vi "get Spectra.vi"() -> ()   [LabVIEW 2020, in "FT-IR.lvlib" / "Get Spectra.lvlib"]
uses:
  Get Spectra.lvlib
  FTIR Diag.ctl
  Aktion FGV Background-Daten.ctl
  FGV FT-IR Diagnose Aktionen.ctl
  Allgemein/allgemeine Sub-VIs.lvlib
  FT-IR.lvlib
panel:
  out "Zeitstempel GB":timestamp caption="Timestamp GoldenBackground" format="%<%x>T"
  in  "GoldenBackground erzeugen":bool caption="Stopp"
  out "DiagLabels":string[](array[string])=["igramdc", "igrampp", "phaseAngle", "laserpp", "laserdc", "badscan", "centerburst", "linCheck", "sBeamIntensity"]
  out "Diagnosewerte für Backup":sgl[](array[numeric])
  out "Zeitstempel":timestamp caption="Timestamp Reference"
  in  "Referenz":bool
  in  "@2500":bool
  in  "FTIR Diag":T1 items=["Background Igram", "Background sBeam", "sample Igram", "sample Background", "sample Absorbance"]
  out "XY-Graph":cluster{"Ramp Pattern":dbl[], dbl[]}[](graph)
  in  "Stopp":bool
  # "FT-IR Diagnose"
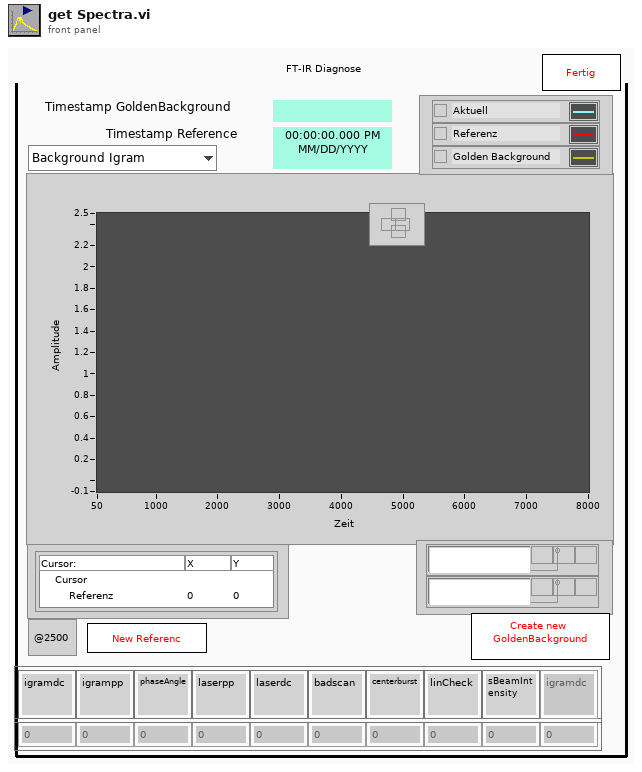
[diagram p1: front panel]
types:
  T1 = typedef "FT-IR.lvlib/Get Spectra.lvlib/FTIR Diag.ctl" = u16
  T2 = typedef "FT-IR.lvlib/Get Spectra.lvlib/Aktion FGV Background-Daten.ctl" = enum16{"lesen", "schreiben", "Background aktiv", "Referenz", "laden", "speichern", "Plot sichtbar"}
  T3 = typedef "FT-IR.lvlib/FGV FT-IR Diagnose Aktionen.ctl" = enum16{"Lesen", "Diagnose Schreiben", "Min Schreiben", "Max Schreiben"}
  T4 = typedef "FT-IR.lvlib/TOOLweb Interface.lvlib/Typdefinitionen.lvlib/TOOLweb Diagnose.ctl" = cluster{"(14) temperature":sgl, "(15) pressure":sgl, "(16) oxygen":sgl, "(50) diag-igramdc":sgl, "(51) diag-igrampp":sgl, "(52) diag-phaseAngle":sgl, "(53) diag-laserpp":sgl, "(54) diag-laserdc":sgl, "(55) diag-badscan":sgl, "(56) diag-centerburst":sgl, "(57) diag-linearizerCheck":sgl, "(58) diag-SNR":sgl, "(59) diag-sBeamIntensity":sgl}
  T5 = typedef "LVPositionTypeDef.ctl" = cluster{"Left":i32, "Top":i32}
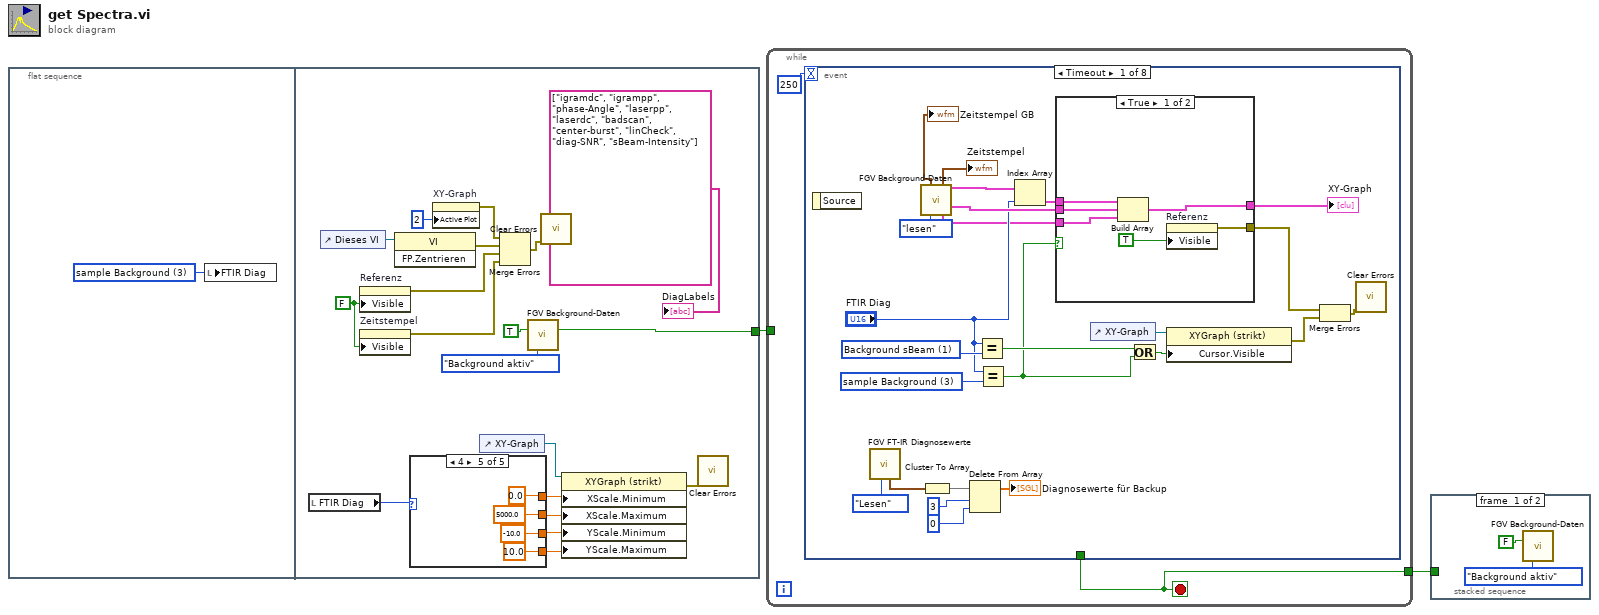
[diagram p0: block diagram]
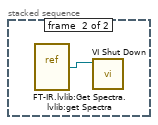
[diagram p2: hidden frame]
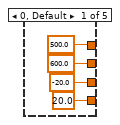
[diagram p3: hidden frame]
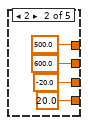
[diagram p4: hidden frame]
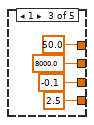
[diagram p5: hidden frame]
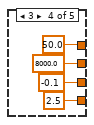
[diagram p6: hidden frame]
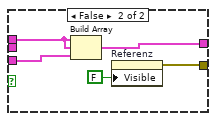
[diagram p7: hidden frame]
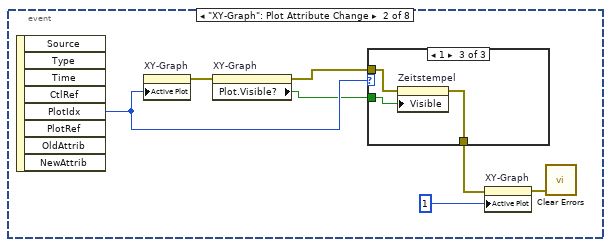
[diagram p8: hidden frame]
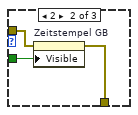
[diagram p10: hidden frame]
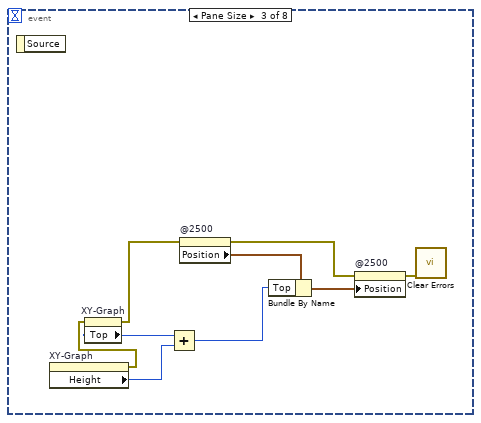
[diagram p11: hidden frame]
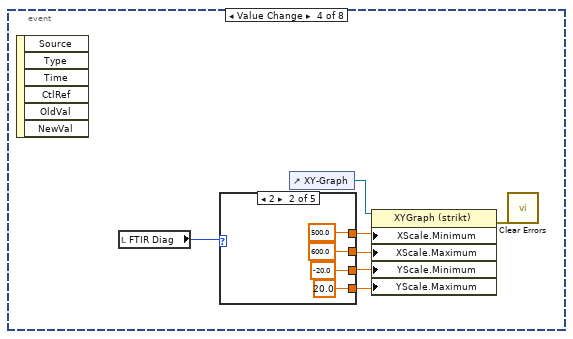
[diagram p12: hidden frame]
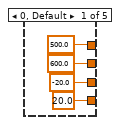
[diagram p13: hidden frame]
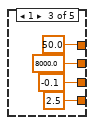
[diagram p14: hidden frame]
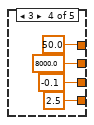
[diagram p15: hidden frame]
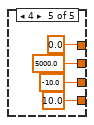
[diagram p16: hidden frame]
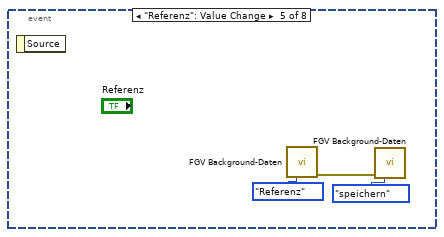
[diagram p17: hidden frame]
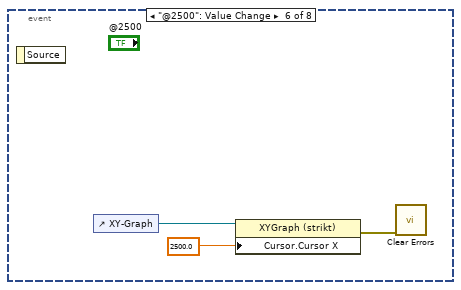
[diagram p18: hidden frame]
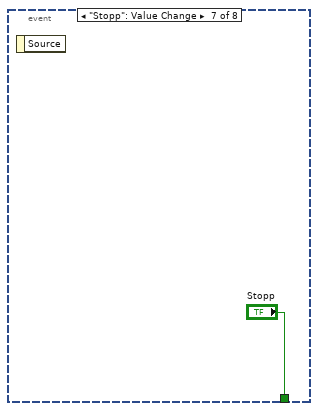
[diagram p19: hidden frame]
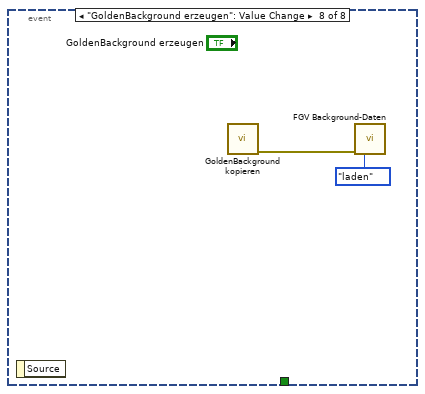
[diagram p20: hidden frame]
diagram:
  n1 = flat-sequence {
    tunnel: [w20] -> w1
    frame #0 {
      w3 = T1 3 items=["Background Igram", "Background sBeam", "sample Igram", "sample Background", "sample Absorbance"] ("FTIR Diag")
      n2 = local write "FTIR Diag"(w3) -> ()
    }
    frame #1 {
      w13 = FALSE ("Sichtbar")
      n3 = local read "FTIR Diag"() -> (w5:T1)
      n4 = control-ref of="Dieses VI"() -> (w19:refnum<vi>)
      n5 = property on="Referenz" class="Bool."("Visible"=w13) -> (error out=w14:errorcluster)  [unwired: 2 in, 1 out]
      n6 = property on="Zeitstempel" class="AbsZeit (strikt)"("Visible"=w13) -> (error out=w12:errorcluster)  [unwired: 2 in, 1 out]
      n7 = invoke class="VI" method="FP.Zentrieren"(reference=w19) -> (error out=w17:errorcluster)  [unwired: 2 in, 2 out]
      n8 = case shown="4" w5 {
        tunnel: [500.0 ("X-Achse.Bereich:Minimum") 500.0 ("X-Achse.Bereich:Minimum") 50.0 ("X-Achse.Bereich:Minimum") 50.0 ("X-Achse.Bereich:Minimum") 0.0 ("X-Achse.Bereich:Minimum")] -> w9
        tunnel: [600.0 ("X-Achse.Bereich:Minimum") 600.0 ("X-Achse.Bereich:Minimum") 8000.0 ("X-Achse.Bereich:Minimum") 8000.0 ("X-Achse.Bereich:Minimum") 5000.0 ("X-Achse.Bereich:Minimum")] -> w8
        tunnel: [-20.0 ("X-Achse.Bereich:Minimum") -20.0 ("X-Achse.Bereich:Minimum") -0.1 ("X-Achse.Bereich:Minimum") -0.1 ("X-Achse.Bereich:Minimum") -10.0 ("X-Achse.Bereich:Minimum")] -> w10
        tunnel: [20.0 ("X-Achse.Bereich:Minimum") 20.0 ("X-Achse.Bereich:Minimum") 2.5 ("X-Achse.Bereich:Minimum") 2.5 ("X-Achse.Bereich:Minimum") 10.0 ("X-Achse.Bereich:Minimum")] -> w11
        frame 0, Default {
        }
        frame 2 {
        }
        frame 1 {
        }
        frame 3 {
        }
        frame 4 {
        }
      }
      n9 = property on="XY-Graph" class="XYGraph (strikt)"("Active Plot"=u32 2 ("Aktiver Plot")) -> (error out=w16:errorcluster)  [unwired: 2 in, 1 out]
      n10 = control-ref of="XY-Graph"() -> (w7:refnum<vi>)
      n11 = Merge Errors(w16, w17, w14, w12) -> (w15:errorcluster)
      n12 = call "FGV Background-Daten.vi"("Background aktiv"=TRUE, "Aktion"=Aktion_FGV_Background-Daten."Background aktiv") -> ("Background aktiv"=w20:bool)  [unwired: 6 in, 7 out]
      n13 = call <vilib>:"Clear Errors.vi"("error in (no error)"=w15) -> ()  [unwired: 5 in, 2 out]
      n14 = property class="XYGraph (strikt)"(reference=w7, "XScale.Minimum"=w9, "XScale.Maximum"=w8, "YScale.Minimum"=w10, "YScale.Maximum"=w11) -> (error out=w6:errorcluster)  [unwired: 1 in, 1 out]
      n15 = call <vilib>:"Clear Errors.vi"("error in (no error)"=w6) -> ()  [unwired: 5 in, 2 out]
      "DiagLabels" <- string[] ["igramdc", "igrampp", "phase-Angle", "laserpp", "laserdc", "badscan", "center-burst", "linCheck", "diag-SNR", "sBeam-Intensity"]
    }
  }
  n16 = while {
    tunnel: [w43] -> w2
    tunnel: w1 -> [_]
    stop <- w43 stop-if-true
    n17 = event shown="[0] Timeout" {
      selector: _ -> [_ _ _ _ _ _ _ _]
      dyn-events: _ -> [_ _ _ _ _ _ _ _]
      timeout: 250 -> [_ _ _ _ _ _ _ _]
      tunnel: [_ _ _ _ _ _ "Stopp" _] -> w43
      event Timeout {
        w64 = T1 3 items=["Background Igram", "Background sBeam", "sample Igram", "sample Background", "sample Absorbance"] ("y")
        w65 = T1 1 items=["Background Igram", "Background sBeam", "sample Igram", "sample Background", "sample Absorbance"] ("y")
        n18 = event-data() -> ()  [unwired: 1 in, 1 out]
        n19 = call "FGV FT-IR Diagnosewerte.vi"("Aktionen"=FGV_FT-IR_Diagnose_Aktionen."Lesen") -> ("Diagnose mean"=w47:T4)  [unwired: 5 in, 5 out]
        n20 = call "FGV Background-Daten.vi"("Aktion"=Aktion_FGV_Background-Daten."lesen") -> ("Zeitstempel GB"=→"Zeitstempel GB":timestamp, "Zeitstempel"=→"Zeitstempel":timestamp, "Background Daten"=w67:cluster{"Ramp Pattern":dbl[], dbl[]}[], "Referenz"=w60:cluster{"Ramp Pattern":dbl[], dbl[]}, "Golden Background"=w46:cluster{dbl[], "[Y]":sgl[]})  [unwired: 7 in, 3 out]
        n21 = Cluster To Array(cluster=w47) -> (array=w51:sgl[])
        n22 = Delete From Array(array=w51, length=3 ("Länge"), index=0 ("Index")) -> (array with subset deleted=→"Diagnosewerte für Backup":sgl[])  [unwired: 1 out]
        n23 = Equal?(x="FTIR Diag", y=w65) -> (x = y?=w63:bool)
        n24 = Equal?(x="FTIR Diag", y=w64) -> (x = y?=w58:bool)
        n25 = Index Array(array=w67, index="FTIR Diag") -> (element=w61:cluster{"Ramp Pattern":dbl[], dbl[]})
        n26 = case shown="True" w58 {
          tunnel: w61 -> [w74 w78]
          tunnel: w60 -> [w73 _]
          tunnel: [w72 w79] -> w59
          tunnel: [w71 w77] -> w55
          tunnel: w46 -> [w69 w75]
          frame True {
            n27 = Build Array(w74, w73, w69) -> (w72:cluster{"Ramp Pattern":dbl[], "[Y]":dbl[]}[])
            n28 = property on="Referenz" class="Bool."("Visible"=TRUE ("Sichtbar")) -> (error out=w71:errorcluster)  [unwired: 2 in, 1 out]
          }
          frame False {
            n29 = Build Array(w78, w78, w75) -> (w79:cluster{"Ramp Pattern":dbl[], "[Y]":dbl[]}[])
            n30 = property on="Referenz" class="Bool."("Visible"=FALSE ("Sichtbar")) -> (error out=w77:errorcluster)  [unwired: 2 in, 1 out]
          }
        }
        "XY-Graph" <- w59
        n31 = control-ref of="XY-Graph"() -> (w66:refnum<vi>)
        n32 = Or(x=w63, y=w58) -> (x .or. y?=w62:bool)
        n33 = property class="XYGraph (strikt)"(reference=w66, "Cursor.Visible"=w62) -> (error out=w57:errorcluster)  [unwired: 1 in, 1 out]
        n34 = Merge Errors(w55, w57) -> (w56:errorcluster)
        n35 = call <vilib>:"Clear Errors.vi"("error in (no error)"=w56) -> ()  [unwired: 5 in, 2 out]
      }
      event "XY-Graph": Plot Attribute Change {
        n36 = event-data() -> ("PlotIdx"=w86:i32)  [unwired: 1 in, 7 out]
        n37 = property on="XY-Graph" class="XYGraph (strikt)"("Active Plot"=w86) -> (error out=w85:errorcluster)  [unwired: 2 in, 1 out]
        n38 = property on="XY-Graph" class="XYGraph (strikt)"(error in=w85) -> (error out=w84:errorcluster, "Plot.Visible?"=w83:bool)  [unwired: 1 in, 1 out]
        n39 = case shown="1" w86 {
          tunnel: w84 -> [w87 w90 w92]
          tunnel: w83 -> [_ w89 w91]
          tunnel: [w87 w88 w93] -> w81
          frame 0, Default {
          }
          frame 2 {
            n40 = property on="Zeitstempel GB" class="AbsZeit (strikt)"(error in=w90, "Visible"=w89) -> (error out=w88:errorcluster)  [unwired: 1 in, 1 out]
          }
          frame 1 {
            n41 = property on="Zeitstempel" class="AbsZeit (strikt)"(error in=w92, "Visible"=w91) -> (error out=w93:errorcluster)  [unwired: 1 in, 1 out]
          }
        }
        n42 = property on="XY-Graph" class="XYGraph (strikt)"(error in=w81, "Active Plot"=1 ("Plotindex")) -> (error out=w80:errorcluster)  [unwired: 1 in, 1 out]
        n43 = call <vilib>:"Clear Errors.vi"("error in (no error)"=w80) -> ()  [unwired: 5 in, 2 out]
      }
      event Pane Size {
        n44 = event-data() -> ()  [unwired: 1 in, 1 out]
        n45 = property on="XY-Graph" class="XYGraph (strikt)"() -> (error out=w96:errorcluster, "Height"=w102:u32)  [unwired: 2 in, 1 out]
        n46 = property on="XY-Graph" class="XYGraph (strikt)"(error in=w96) -> (error out=w97:errorcluster, "Top"=w98:i32)  [unwired: 1 in, 1 out]
        n47 = Add(x=w98, y=w102) -> (x+y=w99:u32)
        n48 = property on="@2500" class="Bool."(error in=w97) -> (error out=w95:errorcluster, "Position"=w101:T5)  [unwired: 1 in, 1 out]
        n49 = Bundle By Name(cluster=w101, "Top"=w99) -> (w100:T5)
        n50 = property on="@2500" class="Bool."(error in=w95, "Position"=w100) -> (error out=w94:errorcluster)  [unwired: 1 in, 1 out]
        n51 = call <vilib>:"Clear Errors.vi"("error in (no error)"=w94) -> ()  [unwired: 5 in, 2 out]
      }
      event Value Change {
        n52 = event-data() -> ()  [unwired: 1 in, 6 out]
        n53 = local read "FTIR Diag"() -> (w109:T1)
        n54 = case shown="2" w109 {
          tunnel: [500.0 ("X-Achse.Bereich:Minimum") 500.0 ("X-Achse.Bereich:Minimum") 50.0 ("X-Achse.Bereich:Minimum") 50.0 ("X-Achse.Bereich:Minimum") 0.0 ("X-Achse.Bereich:Minimum")] -> w105
          tunnel: [600.0 ("X-Achse.Bereich:Minimum") 600.0 ("X-Achse.Bereich:Minimum") 8000.0 ("X-Achse.Bereich:Minimum") 8000.0 ("X-Achse.Bereich:Minimum") 5000.0 ("X-Achse.Bereich:Minimum")] -> w106
          tunnel: [-20.0 ("X-Achse.Bereich:Minimum") -20.0 ("X-Achse.Bereich:Minimum") -0.1 ("X-Achse.Bereich:Minimum") -0.1 ("X-Achse.Bereich:Minimum") -10.0 ("X-Achse.Bereich:Minimum")] -> w104
          tunnel: [20.0 ("X-Achse.Bereich:Minimum") 20.0 ("X-Achse.Bereich:Minimum") 2.5 ("X-Achse.Bereich:Minimum") 2.5 ("X-Achse.Bereich:Minimum") 10.0 ("X-Achse.Bereich:Minimum")] -> w103
          frame 0, Default {
          }
          frame 2 {
          }
          frame 1 {
          }
          frame 3 {
          }
          frame 4 {
          }
        }
        n55 = control-ref of="XY-Graph"() -> (w107:refnum<vi>)
        n56 = property class="XYGraph (strikt)"(reference=w107, "XScale.Minimum"=w105, "XScale.Maximum"=w106, "YScale.Minimum"=w104, "YScale.Maximum"=w103) -> (error out=w108:errorcluster)  [unwired: 1 in, 1 out]
        n57 = call <vilib>:"Clear Errors.vi"("error in (no error)"=w108) -> ()  [unwired: 5 in, 2 out]
      }
      event "Referenz": Value Change {
        n58 = event-data() -> ()  [unwired: 1 in, 1 out]
        n59 = call "FGV Background-Daten.vi"("Aktion"=Aktion_FGV_Background-Daten."Referenz") -> ("error out"=w130:errorcluster)  [unwired: 7 in, 7 out]
        n60 = call "FGV Background-Daten.vi"("error in (no error)"=w130, "Aktion"=Aktion_FGV_Background-Daten."speichern") -> ()  [unwired: 6 in, 8 out]
      }
      event "@2500": Value Change {
        n61 = event-data() -> ()  [unwired: 1 in, 1 out]
        n62 = control-ref of="XY-Graph"() -> (w134:refnum<vi>)
        n63 = property class="XYGraph (strikt)"(reference=w134, "Cursor.Cursor X"=2500.0 ("Cursor.Cursor-Position:Cursor X")) -> (error out=w135:errorcluster)  [unwired: 1 in, 1 out]
        n64 = call <vilib>:"Clear Errors.vi"("error in (no error)"=w135) -> ()  [unwired: 5 in, 2 out]
      }
      event "Stopp": Value Change {
        n65 = event-data() -> ()  [unwired: 1 in, 1 out]
      }
      event "GoldenBackground erzeugen": Value Change {
        n66 = event-data() -> ()  [unwired: 1 in, 1 out]
        n67 = call "GoldenBackground kopieren.vi"() -> ("error out"=w138:errorcluster)  [unwired: 15 in]
        n68 = call "FGV Background-Daten.vi"("error in (no error)"=w138, "Aktion"=Aktion_FGV_Background-Daten."laden") -> ()  [unwired: 6 in, 8 out]
      }
    }
  }
  n69 = stacked-sequence {
    tunnel: w2 -> [_ _]
    frame #0 {
      n70 = call "FGV Background-Daten.vi"("Background aktiv"=FALSE, "Aktion"=Aktion_FGV_Background-Daten."Background aktiv") -> ()  [unwired: 6 in, 8 out]
    }
    frame #1 {
      n71 = vi-ref "FT-IR.lvlib:Get Spectra.lvlib:get Spectra.vi"() -> (w141:refnum<vi>)
      n72 = call "VI Shut Down.vi"("VI Referenz"=w141) -> ()  [unwired: 11 in]
    }
  }
